vi "PublicMethod Filter.vi"(8 "Full Method Name":string, 11 "error in (no error)":errorcluster) -> (0 "Full Method Name dup":string, 1 "Include?":bool, 3 "error out":errorcluster, 5 "Method Name":string)   [LabVIEW 2019, in "Registry-SMO.lvclass"]
doc: "JKI State Machine Objects (SMO) 1.3.0.56\nJKI - JKI\nCopyright (c) 2017, JKI"
uses:
  Registry-SMO.lvclass
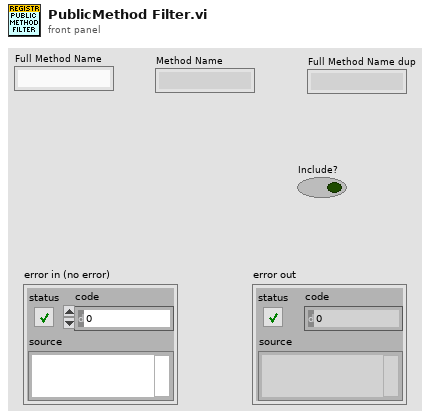
[diagram p1: front panel]
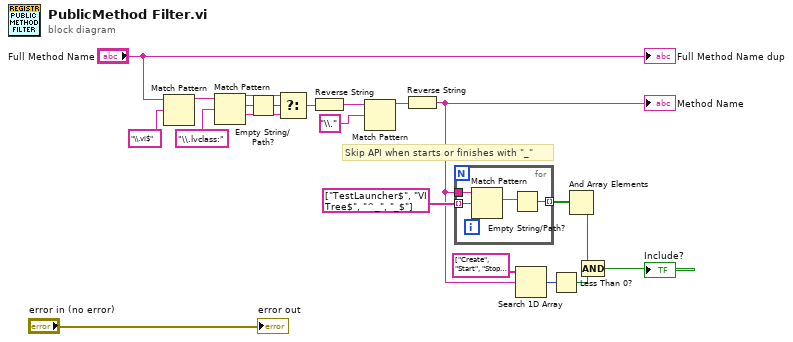
[diagram p0: block diagram]
diagram:
  # "Skip API when starts or finishes with \"_\""
  n1 = Match Pattern(string="Full Method Name", regular expression="\\.vi$") -> (before substring=w8:string)  [unwired: 1 in, 3 out]
  n2 = Match Pattern(string=w8, regular expression="\\.lvclass:") -> (before substring=w4:string, match substring=w6:string, after substring=w3:string)  [unwired: 1 in, 1 out]
  n3 = Empty String/Path?(string/path=w6) -> (empty?=w5:bool)
  n4 = Select(t=w4, s=w5, f=w3) -> (s? t:f=w13:string)
  n5 = Reverse String(1:w13) -> (0:w10:string)
  n6 = Match Pattern(string=w10, regular expression="\\.") -> (before substring=w12:string)  [unwired: 1 in, 3 out]
  n7 = Reverse String(1:w12) -> (0:w19:string)
  "Method Name" <- w19
  n8 = for {
    tunnel: w19 -> [w25]
    tunnel: string[] ["TestLauncher$", "VI Tree$", "^_", "_$"] -> [w24] mode=indexing
    tunnel: [w22] -> w18 mode=indexing
    n9 = Match Pattern(string=w25, regular expression=w24) -> (match substring=w23:string)  [unwired: 1 in, 3 out]
    n10 = Empty String/Path?(string/path=w23) -> (empty?=w22:bool)
  }
  n11 = Search 1D Array(1D array=string[] ["Create", "Start", "Stop", "Destroy", "Get PublicEventRegistration"], element=w19) -> (index of element=w14:i32)  [unwired: 1 in]
  n12 = Less Than 0?(x=w14) -> (x < 0?=w16:bool)
  n13 = And Array Elements(Boolean array=w18) -> (logical AND=w21:bool)
  n14 = Compound Arithmetic op=AND(w21, w16) -> (→"Include?":bool)
  "Full Method Name dup" <- "Full Method Name"
  "error out" <- "error in (no error)"
